vi "CSM - Global Log Queue Monitoring Loop.vi"() -> ()   [LabVIEW 2017, in "CSM-QuickDrops.lvlib"]
uses:
  CSM-QuickDrops.lvlib
  Utility/_support/Periodic String Filter Level.ctl
  Utility/Periodic String Filter Setting.ctl
  Communicable State Machine.lvlib
  _Shared/CSM Shared.lvlib
panel:
  in  "Stop":bool
  out "Level":T1
  out "LogInQ change(#/s)":dbl
  out "log handling Speed(#/s)":dbl
  out "LogInQ":i32
  out "State History":string
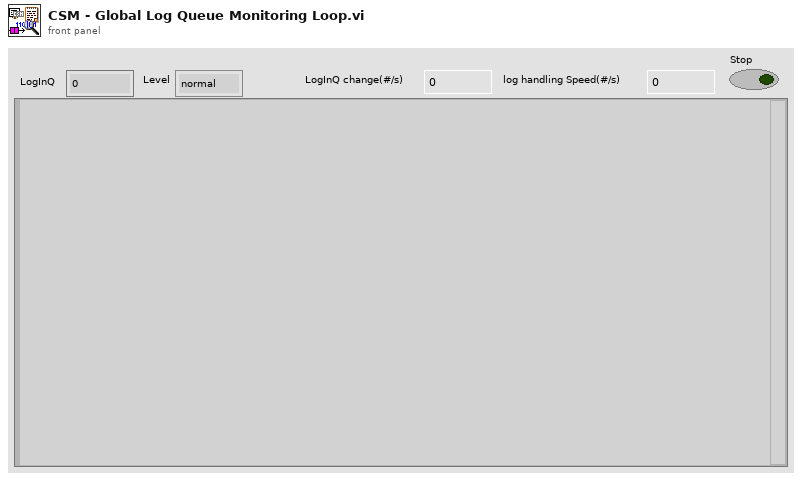
[diagram p1: front panel]
types:
  T1 = typedef "Communicable State Machine.lvlib/Periodic String Filter Level.ctl" = enum16{"normal", "L1", "L2", "L3", "L4"}
  T2 = typedef "Communicable State Machine.lvlib/Periodic String Filter Setting.ctl" = cluster{"threashold(#/s)":dbl, "Check Peroid(s)":dbl}
  T3 = typedef "Communicable State Machine.lvlib/_CSM_GlobalLog_MSG.ctl" = cluster{"Name (\"\" to Use UUID)":string, "Current State":string, "Arguments":string, "Source Message":T4, "Source Module":string, "Complete(T)/Start(F)":bool, "LogType":T5, "Time Stamp":timestamp}
  T4 = typedef "Communicable State Machine.lvlib/_CSM_Response Source Message.ctl" = cluster{"‘State":string, "’Arguments":string, "’Error":errorcluster}
  T5 = typedef "Communicable State Machine.lvlib/_CSM_GlobalLog_MSG_TYPE.ctl" = enum16{"User Log", "State Change", "Status", "Interrupt", "Register", "Unregister", "Error Log", "Module Created", "Module Destroyed"}
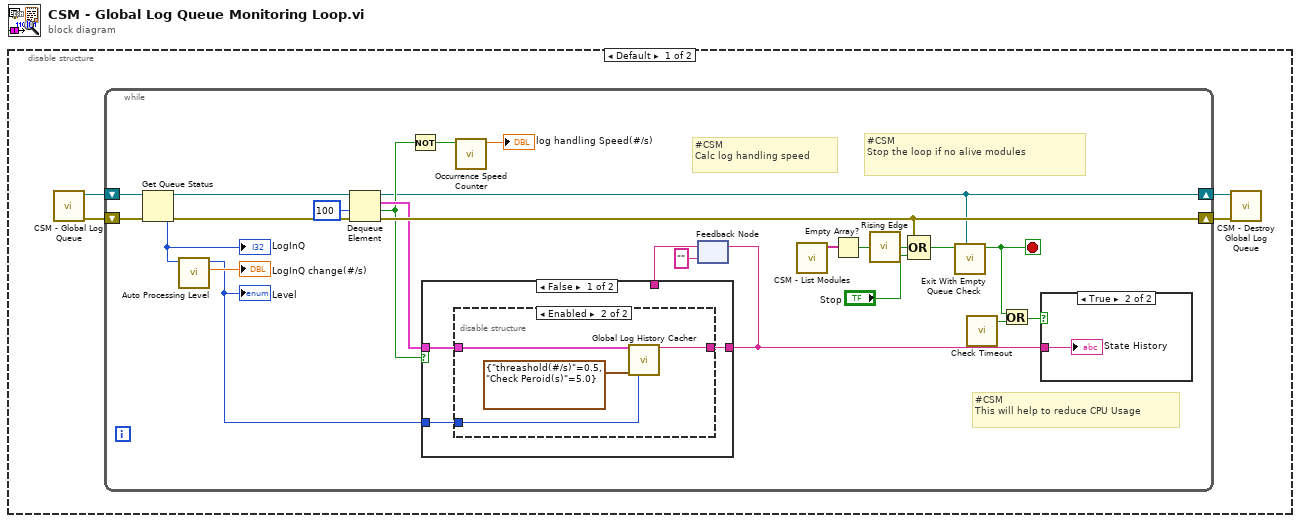
[diagram p0: block diagram]
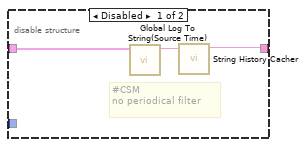
[diagram p2: hidden frame]
diagram:
  n1 = disable-structure shown="Default" {
    frame condition #0 (active) {
      n2 = call "CSM - Global Log Queue.vi"() -> ("error out"=w3:errorcluster, "Global Log Queue"=w1:refnum<queue>)  [unwired: 10 in]
      n3 = while {
        shift-right: [w28] -> w4
        shift-left: w3 -> [w25]
        shift-right: [w12] -> w2
        shift-left: w1 -> [w29]
        stop <- w5 stop-if-true
        # "#CSM\nCalc log handling speed"
        # "#CSM\nStop the loop if no alive modules"
        # "#CSM\nThis will help to reduce CPU Usage"
        n4 = Get Queue Status(queue=w29, error in (no error)=w25) -> (queue out=w27:refnum<queue>, error out=w26:errorcluster, # elements in queue=w8:i32)  [unwired: 1 in, 5 out]
        "LogInQ" <- w8
        n5 = call "Auto Processing Level.vi"("#Left In Q"=w8) -> ("LogInQ Changing Speed (#/s)"=→"LogInQ change(#/s)":dbl, "Level"=w7:T1)  [unwired: 8 in, 1 out]
        "Level" <- w7
        n6 = Dequeue Element(queue=w27, timeout in ms (-1)=100, error in (no error)=w26) -> (queue out=w12:refnum<queue>, element=w24:T3, timed out?=w14:bool, error out=w28:errorcluster)
        n7 = Not(x=w14) -> (.not. x?=w13:bool)
        n8 = call "Occurrence Speed Counter.vi"("Occured? (T)"=w13) -> ("Speed (#/s)"=→"log handling Speed(#/s)":dbl)  [unwired: 8 in, 2 out]
        n9 = feedback #1("" ("String Cache")) -> (w20:string)
        n10 = case shown="False" w14 {
          tunnel: w24 -> [w32 _]
          tunnel: [w31 w40] -> w21
          tunnel: w20 -> [_ w40]
          tunnel: w7 -> [w30 _]
          frame False {
            n11 = disable-structure shown="Enabled" {
              disable-tunnel: w32 -> [w35 w38]
              disable-tunnel: [w33 w39] -> w31
              disable-tunnel: w30 -> [_ w37]
              frame Disabled {
                # "#CSM \nno periodical filter"
                n12 = call "Global Log To String(Source Time).vi"("Log"=w35) -> ("Log String"=w34:string)  [unwired: 9 in]
                n13 = call "String History Cacher.vi"("String"=w34) -> ("String Cache"=w33:string)  [unwired: 10 in]
              }
              frame Enabled {
                n14 = call "Global Log History Cacher.vi"("Global Log Data"=w38, "Settings"=T2 {"threashold(#/s)"=0.5, "Check Peroid(s)"=5.0}, "Level (Normal)"=w37) -> ("String Cache"=w39:string)  [unwired: 12 in]
              }
            }
          }
          frame True {
          }
        }
        n15 = feedback-in #1(w21) -> ()
        n16 = call "CSM - List Modules.vi"() -> ("Module Names"=w19:string[])  [unwired: 10 in, 1 out]
        n17 = Empty Array?(array=w19) -> (empty?=w18:bool)
        n18 = call "Rising Edge.vi"("Signal"=w18) -> ("Rising Edge"=w17:bool)
        n19 = Compound Arithmetic op=OR(w28, w17, "Stop") -> (w10:bool)
        n20 = call "Exit With Empty Queue Check.vi"("Queue"=w12, "Stop"=w10) -> ("Exit"=w5:bool)  [unwired: 8 in, 1 out]
        n21 = call "Check Timeout.vi"() -> ("Timeout"=w22:bool)  [unwired: 8 in]
        n22 = Or(x=w5, y=w22) -> (x .or. y?=w11:bool)
        n23 = case shown="True" w11 {
          tunnel: w21 -> [_ w41]
          frame False {
          }
          frame True {
            "State History" <- w41
          }
        }
      }
      n24 = call "CSM - Destroy Global Log Queue.vi"("Error In"=w4, "Global Log Queue"=w2) -> ()  [unwired: 9 in, 1 out]
    }
    frame condition #1 {
    }
  }
